vi "Calculate Levenshtein Distance.vi"(1 "Pattern":string, 2 "Source":string) -> (0 "Distance":i32)   [LabVIEW 2016, in "Suggestion Box.lvclass"]
doc: "Calculates the Levenshtein <b>Distance</b> between <b>Word</b> and <b>Query</b>, which is a measure of the difference between two sequences of characters.\n--------------------\nCopyright (c) 2019 Analog Devices, Inc. All rights reserved.\n\nRedistribution and use in source and binary forms, with or without modification,\nare permitted provided that the following conditions are met:\n - Redistributions of source code must retain the above copyright notice, this\n list of conditions and the following disclaimer.\n - Redistributions in binary form must reproduce the above copyright notice,\n this list of conditions and the following disclaimer in the documentation\n and/or other materials provided with the distribution.\n - Modified versions of the software must be conspicuously marked as such.\n - This software is licensed solely and exclusively for use with\n processors/products manufactured by or for Analog Devices, Inc.\n - This software may not be combined or merged with other code in any manner\n that would cause the software to become subject to terms and conditions\n which differ from those listed here.\n - Neither the name of Analog Devices, Inc. nor the names of its contributors\n may be used to endorse or promote products derived from this software\n without specific prior written permission.\n - The use of this software may or may not infringe the patent rights of one or\n more patent holders. This license does not release you from the requirement\n that you obtain separate licenses from these patent holders to use this\n software.\n\nTHIS SOFTWARE IS PROVIDED BY ANALOG DEVICES, INC. AND CONTRIBUTORS \"AS IS\" AND\nANY EXPRESS OR IMPLIED WARRANTIES, INCLUDING, BUT NOT LIMITED TO,\nNON-INFRINGEMENT, TITLE, MERCHANTABILITY AND FITNESS FOR A PARTICULAR PURPOSE\nARE DISCLAIMED. IN NO EVENT SHALL ANALOG DEVICES, INC. OR CONTRIBUTORS BE LIABLE\nFOR ANY DIRECT, INDIRECT, INCIDENTAL, SPECIAL, EXEMPLARY, PUNITIVE OR\nCONSEQUENTIAL DAMAGES (INCLUDING, BUT NOT LIMITED TO, DAMAGES ARISING OUT OF\nCLAIMS OF INTELLECTUAL PROPERTY RIGHTS INFRINGEMENT; PROCUREMENT OF SUBSTITUTE\nGOODS OR SERVICES; LOSS OF USE, DATA, OR PROFITS; OR BUSINESS INTERRUPTION)\nHOWEVER CAUSED AND ON ANY THEORY OF LIABILITY, WHETHER IN CONTRACT, STRICT\nLIABILITY, OR TORT (INCLUDING NEGLIGENCE OR OTHERWISE) ARISING IN ANY WAY OUT OF\nTHE USE OF THIS SOFTWARE, EVEN IF ADVISED OF THE POSSIBILITY OF SUCH DAMAGE.\n\n2019-01-10-7CBSD SLA"
uses:
  Suggestion Box.lvclass
panel:
  # "Copyright (c) 2019 Analog Devices, Inc.  All rights reserved.\n\nRedistribution and use in source and binary forms, with or without modification,\nare permitted provided that the following conditions are met:\n  - Redistributions of source code must retain the above copyright notice, this\n    list of conditions and the following disclaimer.\n  - Redistributions in binary form must reproduce the above copyright notice,\n    this list of conditions and the following disclaimer in the documentation\n    and/or other materials provided with the distribution.\n  - Modified versions of the software must be conspicuously marked as such.\n  - This software is licensed solely and exclusively for use with\n    processors/products manufactured by or for Analog Devices, Inc.\n  - This software may not be combined or merged with other code in any manner\n    that would cause the software to become subject to terms and conditions\n    which differ from those listed here.\n  - Neither the name of Analog Devices, Inc. nor the names of its contributors\n    may be used to endorse or promote products derived from this software\n    without specific prior written permission.\n  - The use of this software may or may not infringe the patent rights of one or\n    more patent holders.  This license does not release you from the requirement\n    that you obtain separate licenses from these patent holders to use this\n    software.\n\nTHIS SOFTWARE IS PROVIDED BY ANALOG DEVICES, INC. AND CONTRIBUTORS \"AS IS\" AND\nANY EXPRESS OR IMPLIED WARRANTIES, INCLUDING, BUT NOT LIMITED TO,\nNON-INFRINGEMENT, TITLE, MERCHANTABILITY AND FITNESS FOR A PARTICULAR PURPOSE\nARE DISCLAIMED. IN NO EVENT SHALL ANALOG DEVICES, INC. OR CONTRIBUTORS BE LIABLE\nFOR ANY DIRECT, INDIRECT, INCIDENTAL, SPECIAL, EXEMPLARY, PUNITIVE OR\nCONSEQUENTIAL DAMAGES (INCLUDING, BUT NOT LIMITED TO, DAMAGES ARISING OUT OF\nCLAIMS OF INTELLECTUAL PROPERTY RIGHTS INFRINGEMENT; PROCUREMENT OF SUBSTITUTE\nGOODS OR SERVICES; LOSS OF USE, DATA, OR PROFITS; OR BUSINESS INTERRUPTION)\nHOWEVER CAUSED AND ON ANY THEORY OF LIABILITY, WHETHER IN CONTRACT, STRICT\nLIABILITY, OR TORT (INCLUDING NEGLIGENCE OR OTHERWISE) ARISING IN ANY WAY OUT OF\nTHE USE OF THIS SOFTWARE, EVEN IF ADVISED OF THE POSSIBILITY OF SUCH DAMAGE.\n\n2019-01-10-7CBSD SLA"
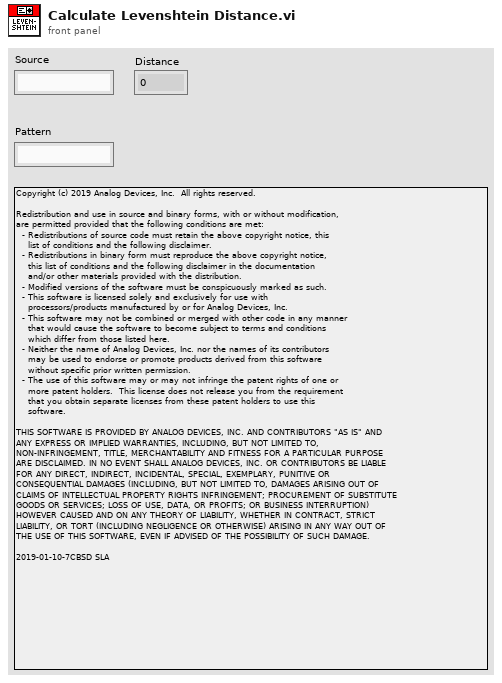
[diagram p1: front panel]
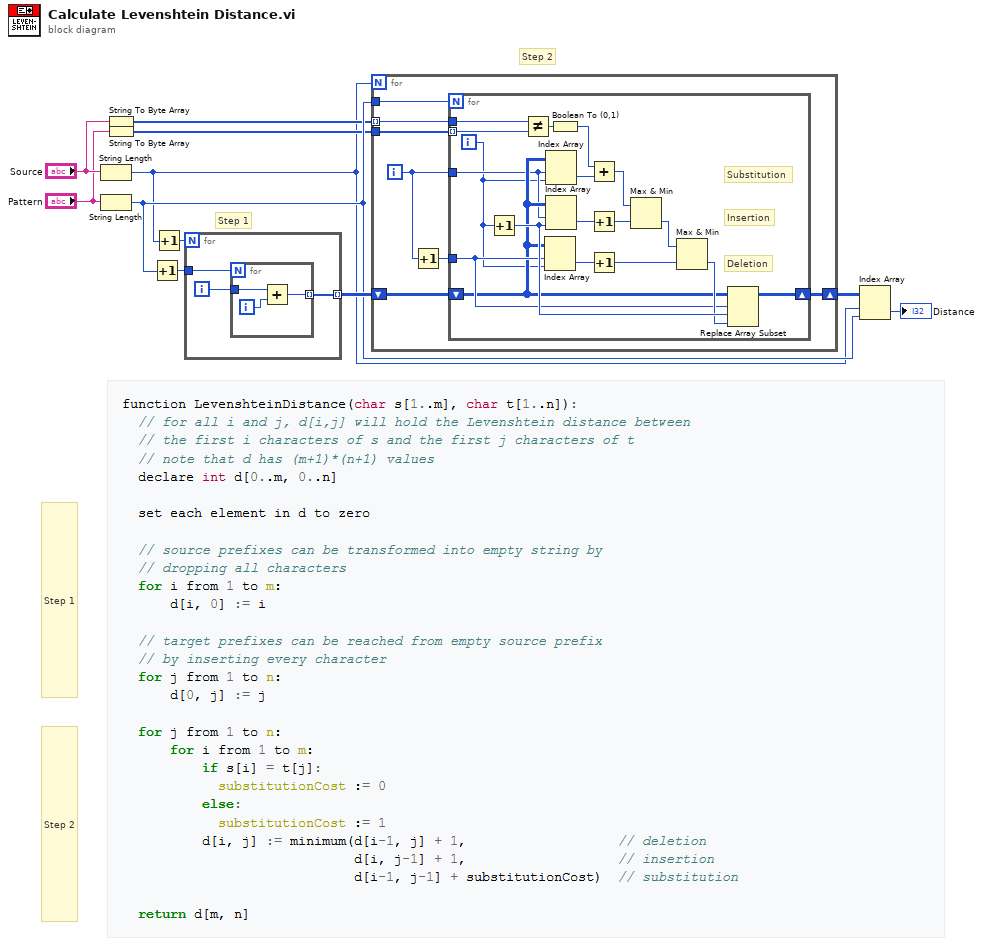
[diagram p0: block diagram]
diagram:
  # "Step 2"
  # "Step 1"
  # "Step 2"
  # "Step 1"
  n1 = String Length(string="Source") -> (length=w1:i32)
  n2 = String Length(string="Pattern") -> (length=w4:i32)
  n3 = String To Byte Array(string="Source") -> (unsigned byte array=w3:u8[])
  n4 = String To Byte Array(string="Pattern") -> (unsigned byte array=w2:u8[])
  n5 = Increment(x=w4) -> (x+1=w6:i32)
  n6 = Increment(x=w1) -> (x+1=w7:i32)
  n7 = for {
    N: w7 -> [_]
    tunnel: w6 -> [w14]
    tunnel: [w12] -> w5 mode=indexing
    i -> [w13]
    n8 = for {
      N: w14 -> [_]
      tunnel: w13 -> [w16]
      tunnel: [w15] -> w12 mode=indexing
      i -> [w17]
      n9 = Add(x=w16, y=w17) -> (x+y=w15:i32)
    }
  }
  n10 = for {
    N: w1 -> [_]
    tunnel: w3 -> [w18] mode=indexing
    tunnel: w2 -> [w24]
    tunnel: w4 -> [w21]
    shift-right: [w19] -> w10
    shift-left: w5 -> [w20]
    i -> [w22]
    n11 = Increment(x=w22) -> (x+1=w23:i32)
    n12 = for {
      N: w21 -> [_]
      tunnel: w18 -> [w41]
      tunnel: w24 -> [w25] mode=indexing
      tunnel: w23 -> [w37]
      tunnel: w22 -> [w28]
      shift-right: [w32] -> w19
      shift-left: w20 -> [w29]
      i -> [w27]
      # "Deletion"
      # "Insertion"
      # "Substitution"
      n13 = Increment(x=w27) -> (x+1=w39:i32)
      n14 = Not Equal?(x=w41, y=w25) -> (x != y?=w40:bool)
      n15 = Index Array(array=w29, index (row)=w37, index (col)=w27) -> (element=w35:i32)
      n16 = Index Array(array=w29, index (row)=w28, index (col)=w27) -> (element=w30:i32)
      n17 = Index Array(array=w29, index (row)=w28, index (col)=w39) -> (element=w36:i32)
      n18 = Boolean To (0,1)(Boolean=w40) -> (0, 1=w31:i16)
      n19 = Add(x=w31, y=w30) -> (x+y=w26:i32)
      n20 = Increment(x=w36) -> (x+1=w34:i32)
      n21 = Increment(x=w35) -> (x+1=w33:i32)
      n22 = Max & Min(x=w26, y=w34) -> (min(x,y)=w42:i32)  [unwired: 1 out]
      n23 = Max & Min(x=w42, y=w33) -> (min(x,y)=w38:i32)  [unwired: 1 out]
      n24 = Replace Array Subset(array=w29, new element=w38, index (row)=w37, index (col)=w39) -> (w32:i32[][])
    }
  }
  n25 = Index Array(array=w10, index (row)=w1, index (col)=w4) -> (element=→"Distance":i32)
